vi "Get Trigger Model Blender Mode.vi"(8 "error in (no error)":errorcluster, 10 "Blender Number (1)":i32=1 format="%#.6g", 11 "VISA resource name":refnum<visa-resource-name>) -> (0 "error out":errorcluster, 2 "Orenable Mode":string, 3 "VISA resource name out":refnum<visa-resource-name>)   [LabVIEW 2020, in "Keithley 2450.lvlib"]
doc: "Returns whether the blender performs OR operations or AND operations."
uses:
  <instrlib>/Keithley 2450/Keithley 2450.lvlib
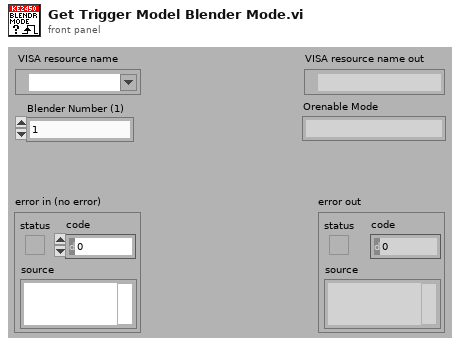
[diagram p1: front panel]
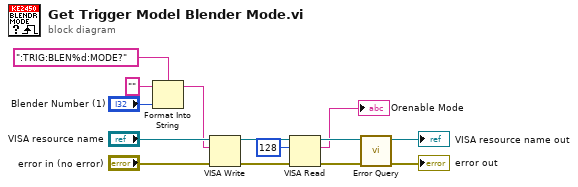
[diagram p0: block diagram]
diagram:
  n1 = Format Into String(format string=":TRIG:BLEN%d:MODE?", initial string="", "Blender Number (1)") -> (resulting string=w7:string)  [unwired: 1 in, 1 out]
  n2 = VISA Write(VISA resource name="VISA resource name", write buffer=w7, error in (no error)="error in (no error)") -> (VISA resource name out=w4:refnum<visa-resource-name>, error out=w6:errorcluster)  [unwired: 1 out]
  n3 = VISA Read(VISA resource name=w4, byte count=u32 128, error in (no error)=w6) -> (VISA resource name out=w3:refnum<visa-resource-name>, read buffer=→"Orenable Mode":string, error out=w5:errorcluster)  [unwired: 1 out]
  n4 = call <instrlib>:"Error Query.vi"("error in (no error)"=w5, "VISA resource name"=w3) -> ("error out"=→"error out":errorcluster, "VISA resource name out"=→"VISA resource name out":refnum<visa-resource-name>)  [unwired: 8 out]
